vi "moisture_project.vi"() -> ()   [LabVIEW 2011]
uses:
  <vilib>/Analysis/NI_AALBase.lvlib
panel:
  out "Standard Deviation\nof Moisture Sensor":dbl format="%0.4f"
  out "Mean of Moisture Sensor (V)":dbl format="%0.4f"
  out "Elapsed Time (sec)":u32 format="%.1f"
  out "Time Response of Sensor":dynamicdata(graph)
  in  "stop (F)":bool
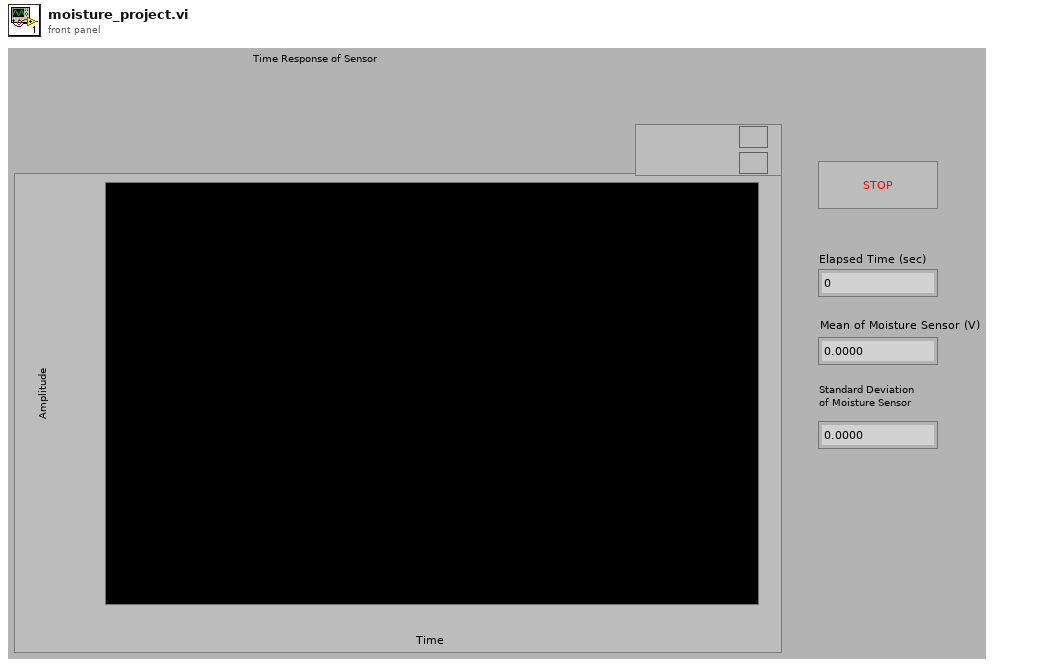
[diagram p1: front panel]
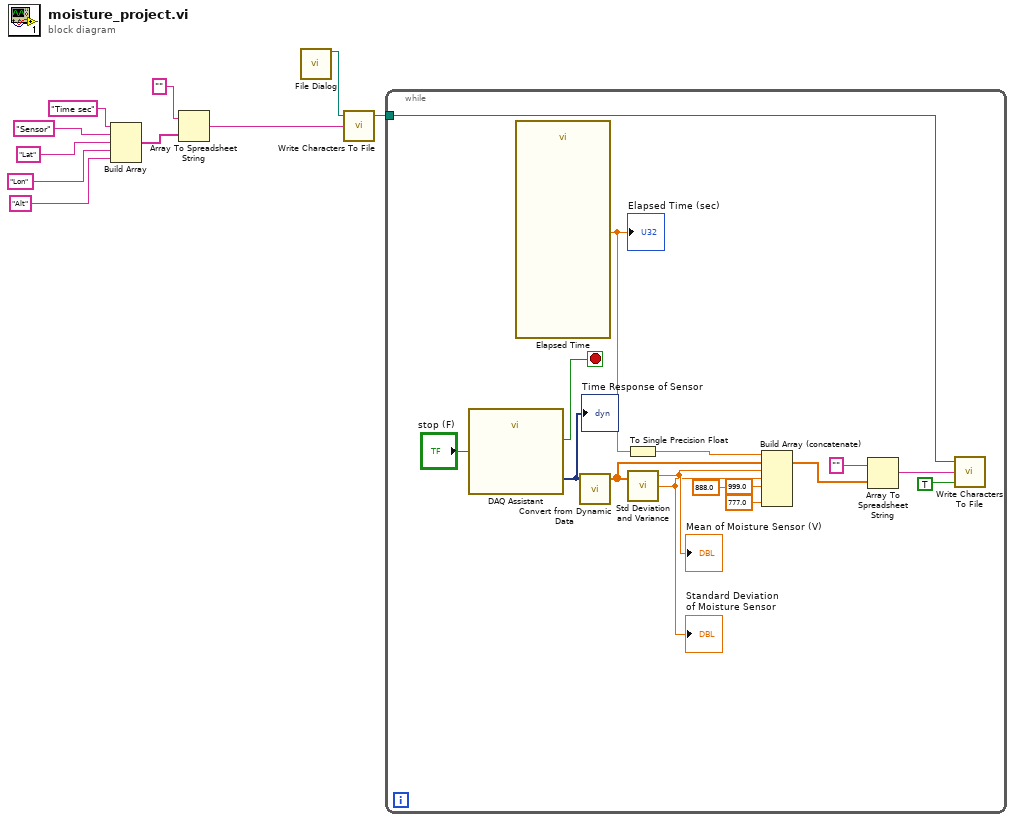
[diagram p0: block diagram]
diagram:
  n1 = Build Array "Build Array"("Time sec" ("element"), "Sensor" ("element"), "Lat" ("element"), "Lon" ("element"), "Alt" ("element")) -> (w6:string[])
  n2 = Array To Spreadsheet String(array=w6, 3:"" ("format string")) -> (spreadsheet string=w9:string)  [unwired: 1 out]
  n3 = call "File Dialog"() -> ("selected path"=w4:path)  [unwired: 7 in, 8 out]
  n4 = call <vilib>:"Write Characters To File.vi"("character string"=w9, "file path (dialog if empty)"=w4) -> ("new file path (Not A Path if cancelled)"=w5:path)  [unwired: 1 in, 2 out]
  n5 = while {
    tunnel: w5 -> [w24]
    stop <- w25 stop-if-true
    n6 = call "DAQ Assistant"("stop (F)"="stop (F)") -> ("data"=w21:dynamicdata, "stopped"=w25:bool)  [unwired: 4 in, 13 out]
    "Time Response of Sensor" <- w21
    n7 = call "Elapsed Time"() -> ("Elapsed Time (s)"=w22:dbl)  [unwired: 5 in, 14 out]
    "Elapsed Time (sec)" <- w22
    n8 = call "Convert from Dynamic Data"("Dynamic Data Type"=w21) -> ("Array"=w20:dbl[])  [unwired: 1 in, 2 out]
    n9 = To Single Precision Float(number=w22) -> (single precision float=w23:sgl)
    n10 = call <vilib>:"Std Deviation and Variance.vi"("X"=w20) -> ("mean"=w16:dbl, "standard deviation"=w15:dbl)  [unwired: 1 in, 1 out]
    "Mean of Moisture Sensor (V)" <- w16
    "Standard Deviation\nof Moisture Sensor" <- w15
    n11 = Build Array (concatenate)(w23, w20, w16, w15, 999.0 ("element"), 888.0 ("element"), 777.0 ("element")) -> (w14:dbl[])
    n12 = Array To Spreadsheet String(array=w14, 3:"" ("format string")) -> (spreadsheet string=w19:string)  [unwired: 1 out]
    n13 = call <vilib>:"Write Characters To File.vi"("append to file? (new file:F)"=TRUE, "character string"=w19, "file path (dialog if empty)"=w24) -> ()  [unwired: 3 out]
  }
